vi "Update Online Status List.vi"(8 "error in (no error)":errorcluster, 10 "User Online Info":T1[](array[typedef]), 11 "Chat Room Model in":refnum<class "Chat Room Model.lvclass">) -> (0 "error out":errorcluster, 3 "Chat Room Model out":refnum<class "Chat Room Model.lvclass">)   [LabVIEW 2020, in "Chat Room Model.lvlib" / "Chat Room Model.lvclass"]
uses:
  Chat Room Model.lvclass
  UI Status Update/User Info.ctl
  Chat Room Model.lvclass/Chat Room Model.ctl
  Chat Window UI Controller/Chat Window UI Controller Messages/Update Online Status List Msg/Update Online Status List Msg.lvclass/Update Online Status List Msg.ctl
  <vilib>/ActorFramework/Message Enqueuer/Message Enqueuer.lvclass/Message Enqueuer.ctl
  <vilib>/ActorFramework/Message Enqueuer/Enqueue.vi
  Chat Window UI Controller/Chat Window UI Controller Messages/Update Online Status List Msg/Update Online Status List Msg.lvclass
  C:/Program Files (x86)/National Instruments/LabVIEW 2020/vi.lib/ActorFramework/Message/Message.lvclass
  <vilib>/ActorFramework/Message Priority Queue/Priority Enqueue.vi
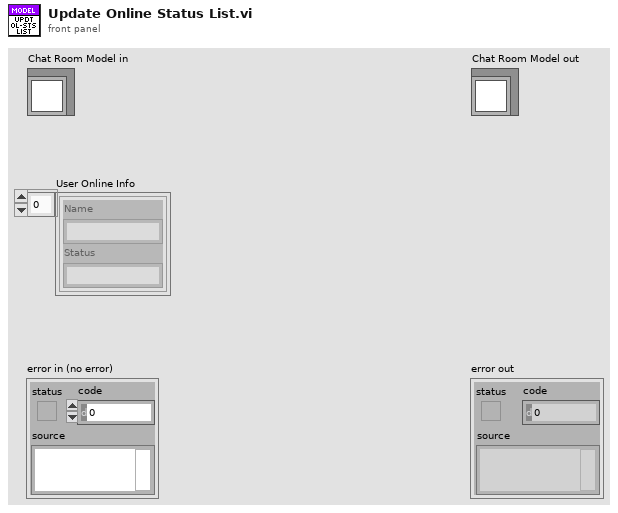
[diagram p1: front panel]
types:
  T1 = typedef "Chat Room Model.lvlib/Chat Room Model.lvclass/User Info.ctl" = cluster{"Name":string, "Status":string}
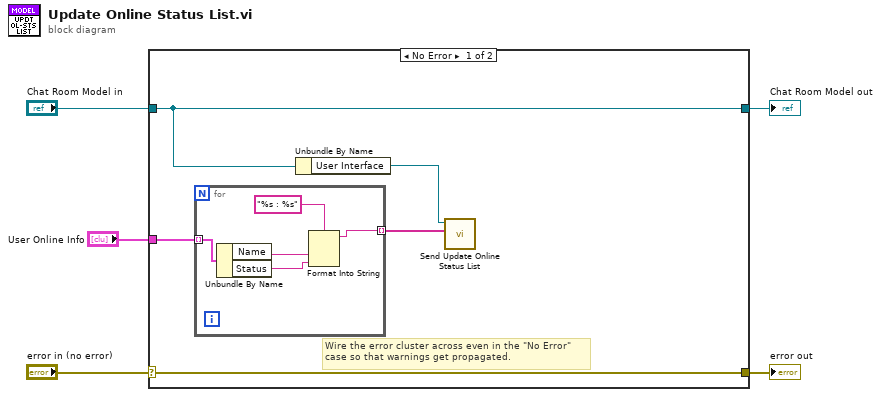
[diagram p0: block diagram]
diagram:
  n1 = case shown="No Error" "error in (no error)" {
    selector: "error in (no error)" -> [w10 w17]
    tunnel: [w10 w17] -> w4
    tunnel: [w9 w16] -> w2
    tunnel: "Chat Room Model in" -> [w9 w16]
    tunnel: "User Online Info" -> [w7 _]
    frame No Error {
      # "Wire the error cluster across even in the \"No Error\"\ncase so that warnings get propagated."
      n2 = for {
        tunnel: w7 -> [w15] mode=indexing
        tunnel: [w11] -> w6 mode=indexing
        n3 = Unbundle By Name(w15) -> ("Name"=w13:string, "Status"=w12:string)
        n4 = Format Into String(format string="%s : %s", w13, w12) -> (resulting string=w11:string)  [unwired: 2 in, 1 out]
      }
      n5 = Unbundle By Name(w9) -> ("User Interface"=w8:refnum<class "Message Enqueuer.lvclass">)
      n6 = call "Send Update Online Status List.vi"("Online Status List"=w6, "Message Enqueuer"=w8) -> ()  [unwired: 8 in, 2 out]
    }
    frame Error {
    }
  }
  "error out" <- w4
  "Chat Room Model out" <- w2
